vi "create collation16.vi"(6 "?":i32, 7 "pArg":u32, 8 "error in (no error)":errorcluster, 9 "eTextRep":i32, 10 "zName":u32, 11 "para0":dbl) -> (0 "error out":errorcluster, 2 "function return":i32, 3 "para0 out":dbl, 5 "pArg out":u32)   [LabVIEW 2020, in "sqlite3.lvlib"]
uses:
  sqlite3.lvlib
  errstr.vi
  bin/sqlite3_64.dll
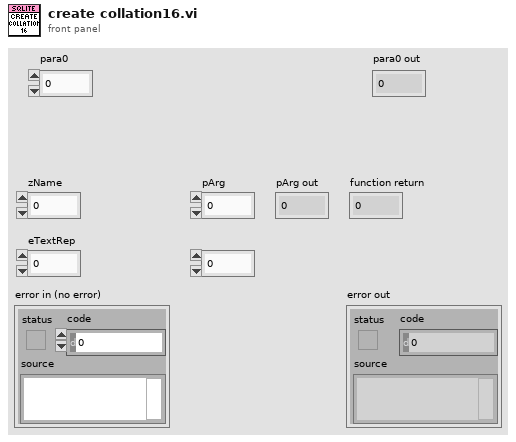
[diagram p1: front panel]
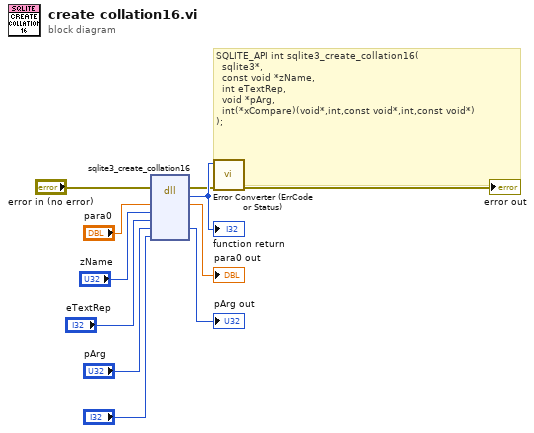
[diagram p0: block diagram]
diagram:
  # "SQLITE_API int sqlite3_create_collation16(\n  sqlite3*, \n  const void *zName,\n  int eTextRep, \n  void *pArg,\n  int(*xCompare)(void*,int,const void*,int,const void*)\n);"
  n1 = dll-call lib="D:/Project/Labview-Projects/database-configuration/externals/sqlite3/Source/bin/sqlite3_*.*" fn="sqlite3_create_collation16"(error in="error in (no error)", "para0"="para0", "zName"="zName", "eTextRep"="eTextRep", "pArg"="pArg", "?") -> (error out=w2:errorcluster, w11:i32, "para0"=→"para0 out":dbl, "pArg"=→"pArg out":u32)  [unwired: 5 in, 1 out]
  "function return" <- w11
  n2 = call "Error Converter (ErrCode or Status).vi"("error in (no error)"=w2, "error code"=w11) -> ("error out"=→"error out":errorcluster)  [unwired: 9 in]
